vi "Quickly light intensity analyze.vi"() -> ()   [LabVIEW 2022 SP3]
uses:
  <vilib>/Math Plots/2D Math Plots/2D Compass/2D Compass XCtrl/2D Compass.xctl
  <vilib>/Analysis/7linalg.llb/Real Transpose Matrix.vi
  <vilib>/Analysis/baseanly.llb/Real A x B.vi
  <vilib>/Analysis/baseanly.llb/A x Vector.vi
  <vilib>/Utility/file.llb/Read Delimited Spreadsheet (DBL).vi
  <vilib>/Analysis/Matrix/Numeric/Conversions/Array To Matrix - RA2.vi
  <vilib>/Analysis/baseanly.llb/Real Inverse Matrix.vi
  <vilib>/Math Plots/2D Math Plots/2D Compass/2D Compass Datatype/Public/Plot Helper (Vector).vi
  <vilib>/Analysis/polynomials.llb/Polynomial Roots (DBL).vi
  <vilib>/Analysis/NI_AALPro.lvlib
  <vilib>/Math Plots/2D Math Plots/2D Compass/2D Compass Datatype/2D Compass Datatype.lvclass
  <vilib>/Math Plots/2D Math Plots/2D Plot/2D Plot Datatype/2D Plot Datatype.lvclass
  <vilib>/Analysis/Matrix/NI_Matrix.lvlib
  <vilib>/Analysis/NI_AALBase.lvlib
panel:
  in  "index":i32
  in  "Psi data base":path=path "C:/Users/User/Desktop/VASE/SiO2_70nm_Psi - 複製.txt"
  in  "Delta data base":path=path "C:/Users/User/Desktop/VASE/SiO2_70nm_Delta - 複製.txt"
  in  "VASE data index AOI35=1 ~AOI65=7":i32=2
  in  "phase retardor":dbl
  out "PSI":dbl
  out "Delta":dbl
  in  "Calculate Psi delta":bool
  out "2D Compass":refnum<class "2D Plot Datatype.lvclass">[](xcontrol)
  out "Intensity Graph 2":dbl[][](graph)
  in  "X :":dbl=1.0
  in  "Square side length:":dbl=511.0
  in  "Y :":dbl=1.0
  out "Max value(fitting)":dbl
  out "Degree exp 2":i32
  out "Max value(exp)":dbl
  in  "多項式fittng之最高次":i32=34
  in  "間隔角度":i32=10
  in  "亮度扣除基底":dbl=500.0 format="%#_13g"
  out "Intensity profile ratial":dbl
  out "all rows":dbl[][](array[numeric])
  out "Degree exp":i32
  out "Min value(exp)":dbl
  out "Min value(fitting)":dbl
  in  "起始角度":i32=10
  out "Pure Complex Roots":cdb[](array[numeric])
  out "Complex Pair Roots":cdb[](array[numeric])
  out "Seconds  2":dbl
  out "Minutes":dbl
  out "Hours  2":dbl
  out "Files currently reading  2":string
  in  "Choose an arbitrary file in the angle of incidence folder :":path
  out "極值位置":dbl[](array[numeric])
  out "Light Intensity":cluster{i32[], "Array":dbl[]}[](graph)
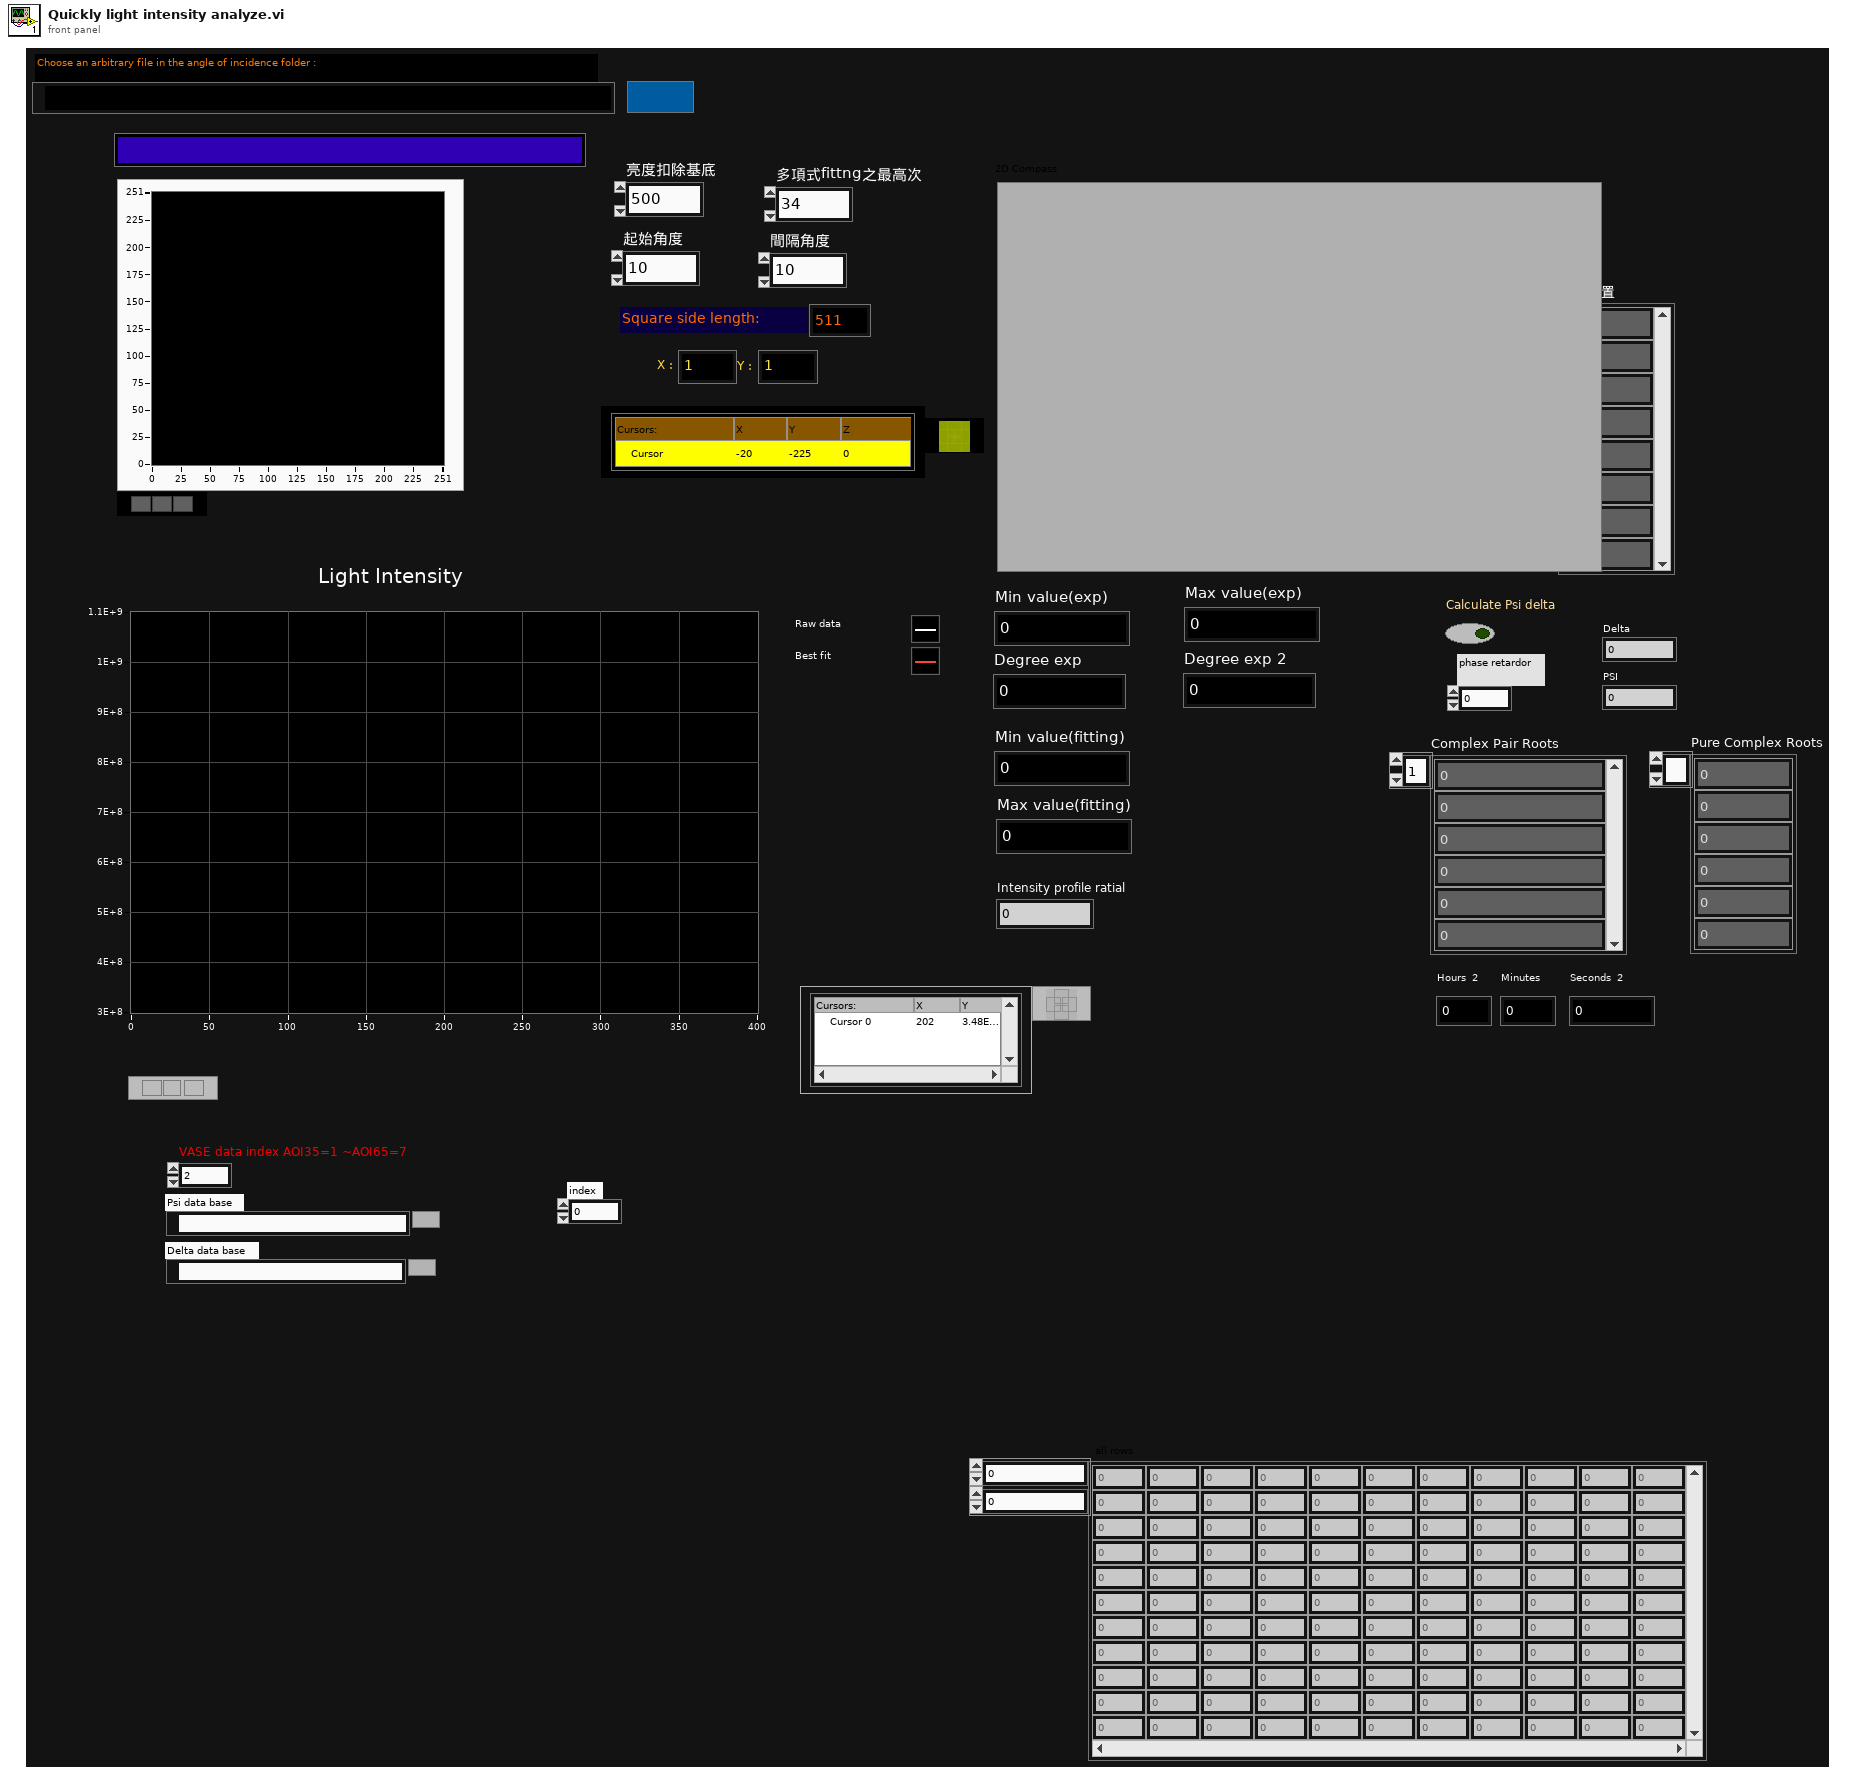
[diagram p1: front panel]
types:
  T1 = typedef "NI_Matrix.lvlib/RealMatrix.ctl" = dbl[][]
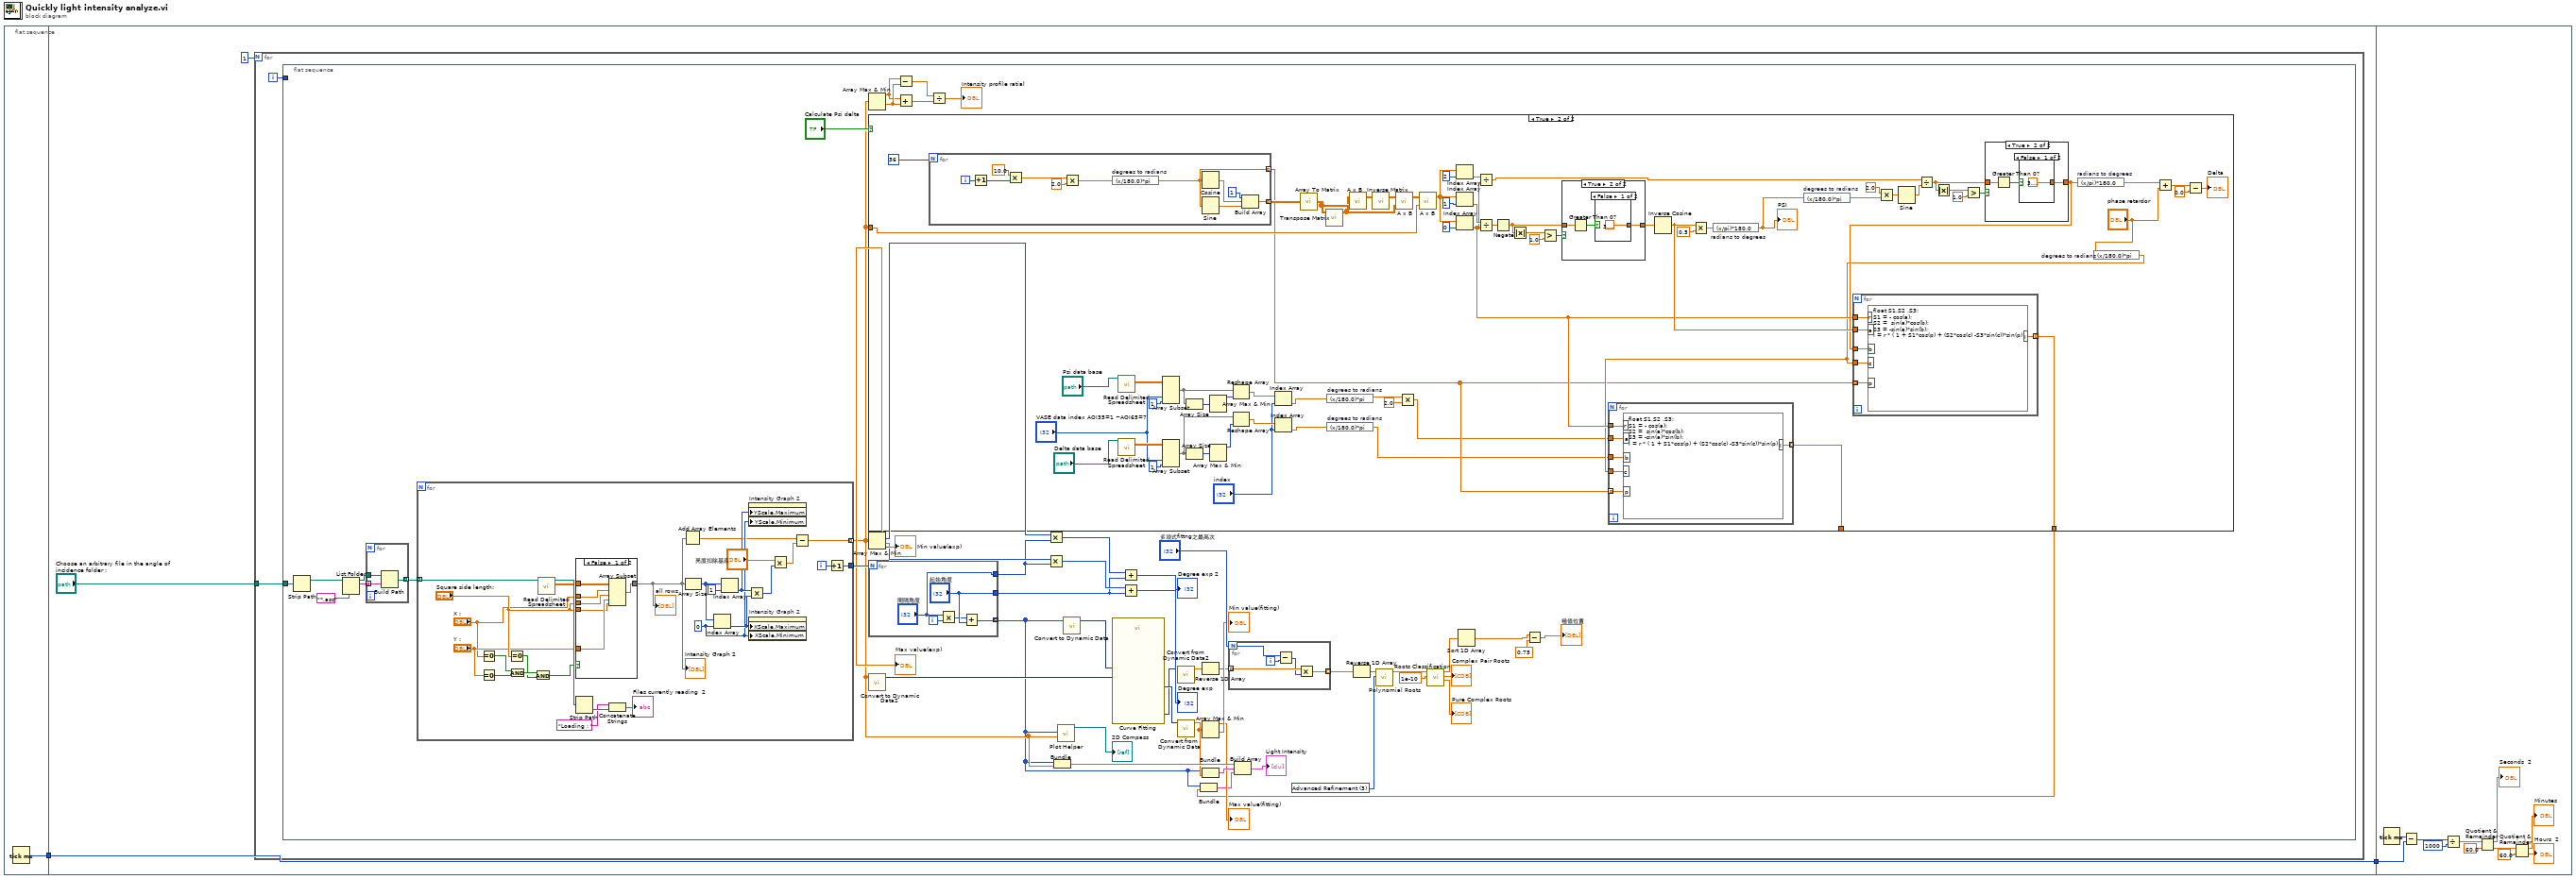
[diagram p0: block diagram]
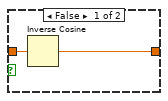
[diagram p3: hidden frame]
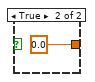
[diagram p4: hidden frame]
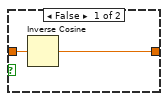
[diagram p5: hidden frame]
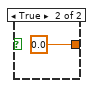
[diagram p6: hidden frame]
diagram:
  n1 = flat-sequence {
    tunnel: [w3] -> w2
    tunnel: [w6] -> w1
    tunnel: w2 -> [w6]
    tunnel: w1 -> [w211]
    frame #0 {
      n2 = Tick Count (ms)() -> (millisecond timer value=w3:u32)
    }
    frame #1 {
      n3 = for {
        N: 1 -> [_]
        tunnel: "Choose an arbitrary file in the angle of incidence folder :" -> [w7]
        i -> [w8]
        n4 = flat-sequence {
          tunnel: w8 -> [_]
          tunnel: w7 -> [w47]
          frame #0 {
            w55 = u16 3 items=["General", "Simple Classification", "Refinement", "Advanced Refinement"] ("option")
            n5 = Strip Path(path=w47) -> (stripped path=w52:path)  [unwired: 1 out]
            n6 = List Folder(path=w52, pattern="*.asc") -> (path out=w51:path, filenames=w50:string[])  [unwired: 2 in, 2 out]
            n7 = for {
              tunnel: w50 -> [w165] mode=indexing
              tunnel: w51 -> [w166]
              tunnel: [w164] -> w48 mode=indexing
              n8 = Build Path(base path=w166, name or relative path=w165) -> (appended path=w164:path)
            }
            n9 = for {
              tunnel: [w178] -> w16 mode=indexing
              tunnel: w48 -> [w199] mode=indexing
              tunnel: [w197] -> w40
              i -> [w198]
              w184 = 0 ("index")
              n10 = Equal To 0?(x="X :") -> (x = 0?=w195:bool)
              n11 = Equal To 0?(x="Y :") -> (x = 0?=w196:bool)
              n12 = Equal To 0?(x="Square side length:") -> (x = 0?=w188:bool)
              n13 = And(x=w195, y=w196) -> (x .and. y?=w194:bool)
              n14 = And(x=w194, y=w188) -> (x .and. y?=w193:bool)
              n15 = call-poly <vilib>:"Read Delimited Spreadsheet.vi"("file path (dialog if empty)"=w199) -> ("new file path (Not A Path if cancelled)"=w200:path, "all rows"=w183:dbl[][])  [unwired: 9 in, 4 out]
              n16 = case shown="False" w193 {
                tunnel: w183 -> [w209 w210]
                tunnel: "X :" -> [w207 _]
                tunnel: "Y :" -> [w206 _]
                tunnel: [w208 w210] -> w177
                tunnel: "Square side length:" -> [w205 _]
                tunnel: "Square side length:" -> [w204 _]
                frame False {
                  n17 = Array Subset(array=w209, index (row)=w207, length (row)=w205, index (col)=w206, length (col)=w204) -> (w208:dbl[][])
                }
                frame True {
                }
              }
              "all rows" <- w177
              "Intensity Graph 2" <- w177
              n18 = Strip Path(path=w200) -> (name=w202:string)  [unwired: 1 out]
              n19 = Concatenate Strings("Loading : " ("string"), w202) -> (→"Files currently reading  2":string)
              n20 = Add Array Elements(numeric array=w177) -> (sum=w182:dbl)
              n21 = Array Size(array=w177) -> (size(s)=w192:i32[])
              n22 = Index Array(array=w192, index=w184) -> (element=w189:i32)
              n23 = Index Array(array=w192, index=1) -> (element=w190:i32)
              n24 = Multiply(x=w190, y=w189) -> (x*y=w181:i32)
              n25 = property on="Intensity Graph 2" class="IntGraph (strict)"("YScale.Maximum"=w190, "YScale.Minimum"=w184) -> ()  [unwired: 2 in, 2 out]
              n26 = property on="Intensity Graph 2" class="IntGraph (strict)"("XScale.Maximum"=w189, "XScale.Minimum"=w184) -> ()  [unwired: 2 in, 2 out]
              n27 = Multiply(x="亮度扣除基底", y=w181) -> (x*y=w179:dbl)
              n28 = Subtract(x=w182, y=w179) -> (x-y=w178:dbl)
              n29 = Increment(x=w198) -> (x+1=w197:i32)
            }
            n30 = Array Max & Min(array=w16) -> (max value=w42:dbl, min value=w43:dbl)  [unwired: 2 out]
            n31 = case shown="True" "Calculate Psi delta" {
              tunnel: w16 -> [_ w112]
              tunnel: [_ w95] -> w14
              tunnel: [_ w83] -> _
              frame False {
              }
              frame True {
                n32 = for {
                  N: 36 ("Numeric") -> [_]
                  tunnel: [w160] -> w119 mode=indexing
                  tunnel: [w153] -> w84 mode=indexing
                  i -> [w163]
                  n33 = Increment(x=w163) -> (x+1=w162:i32)
                  n34 = Multiply(x=10.0, y=w162) -> (x*y=w158:dbl)
                  n35 = Multiply(x=w158, y=2.0) -> (x*y=w154:dbl)
                  n36 = expression code="(x/180.0)*pi" "degrees to radians"(w154) -> (w153:dbl)
                  n37 = Cosine(x=w153) -> (cos(x)=w156:dbl)
                  n38 = Sine(x=w153) -> (sin(x)=w157:dbl)
                  n39 = Build Array(1, w156, w157) -> (w160:dbl[])
                }
                n40 = call-poly <vilib>:"Read Delimited Spreadsheet.vi"("file path (dialog if empty)"="Psi data base") -> ("all rows"=w81:dbl[][])  [unwired: 9 in, 5 out]
                n41 = call-poly <vilib>:"Read Delimited Spreadsheet.vi"("file path (dialog if empty)"="Delta data base") -> ("all rows"=w75:dbl[][])  [unwired: 9 in, 5 out]
                n42 = Array Subset(array=w81, index (col)="VASE data index AOI35=1 ~AOI65=7", length (col)=1 ("length")) -> (w77:dbl[][])  [unwired: 2 in]
                n43 = Array Subset(array=w75, index (col)="VASE data index AOI35=1 ~AOI65=7", length (col)=1 ("length")) -> (w71:dbl[][])  [unwired: 2 in]
                n44 = Array Size(array=w77) -> (size(s)=w79:i32[])
                n45 = Array Size(array=w71) -> (size(s)=w73:i32[])
                n46 = Array Max & Min(array=w79) -> (max value=w78:i32)  [unwired: 3 out]
                n47 = Array Max & Min(array=w73) -> (max value=w72:i32)  [unwired: 3 out]
                n48 = Reshape Array(w77, w78) -> (w69:dbl[])
                n49 = Reshape Array(w71, w72) -> (w68:dbl[])
                n50 = Index Array(array=w69, index="index") -> (element=w66:dbl)
                n51 = Index Array(array=w68, index="index") -> (element=w65:dbl)
                n52 = call-poly <vilib>:"Array To Matrix.vi"("Real 2D Array"=w119) -> ("Real Matrix"=w125:T1)
                n53 = call-poly <vilib>:"Transpose Matrix.vi"("Input Matrix"=w125) -> ("Matrix Transpose"=w122:T1)  [unwired: 9 in, 1 out]
                n54 = expression code="(x/180.0)*pi" "degrees to radians"(w66) -> (w64:dbl)
                n55 = expression code="(x/180.0)*pi" "degrees to radians"(w65) -> (w61:dbl)
                n56 = call-poly <vilib>:"A x B.vi"("B"=w125, "A"=w122) -> ("A x B"=w124:T1)  [unwired: 1 out]
                n57 = call-poly <vilib>:"Inverse Matrix.vi"("Input Matrix"=w124) -> ("Inverse Matrix"=w123:T1)  [unwired: 1 in, 1 out]
                n58 = call-poly <vilib>:"A x B.vi"("B"=w122, "A"=w123) -> ("A x B"=w121:T1)  [unwired: 1 out]
                n59 = Multiply(x=w64, y=2.0) -> (x*y=w62:dbl)
                n60 = call-poly <vilib>:"A x B.vi"("Vector"=w112, "A"=w121) -> ("A x Vector"=w114:dbl[])  [unwired: 1 out]
                n61 = Index Array(array=w114, index=2) -> (element=w113:dbl)
                n62 = Index Array(array=w114, index=1) -> (element=w116:dbl)
                n63 = Index Array(array=w114, index=0) -> (element=w86:dbl)
                n64 = Divide(x=w113, y=w86) -> (x/y=w98:dbl)
                n65 = Divide(x=w116, y=w86) -> (x/y=w115:dbl)
                n66 = Negate(x=w115) -> (-x=w89:dbl)
                n67 = Absolute Value(x=w89) -> (abs(x)=w92:dbl)
                n68 = Greater?(x=w92, y=1.0) -> (0:w90:bool)
                n69 = case shown="True" w90 {
                  tunnel: [w133 w136] -> w88
                  tunnel: w89 -> [w134 w135]
                  frame False {
                    n70 = Inverse Cosine(1:w134) -> (0:w133:dbl)
                  }
                  frame True {
                    n71 = Greater Than 0?(x=w135) -> (x > 0?=w137:bool)
                    n72 = case shown="False" w137 {
                      tunnel: [3.141592653589793 0.0] -> w136
                      frame False {
                      }
                      frame True {
                      }
                    }
                  }
                }
                n73 = Inverse Cosine(1:w88) -> (0:w94:dbl)
                n74 = Multiply(x=w94, y=0.5) -> (x*y=w110:dbl)
                n75 = expression code="(x/pi)*180.0" "radians to degrees"(w110) -> (w99:dbl)
                "PSI" <- w99
                n76 = expression code="(x/180.0)*pi" "degrees to radians"(w99) -> (w104:dbl)
                n77 = Multiply(x=2.0, y=w104) -> (x*y=w102:dbl)
                n78 = Sine(x=w102) -> (sin(x)=w105:dbl)
                n79 = Divide(x=w98, y=w105) -> (x/y=w106:dbl)
                n80 = Absolute Value(x=w106) -> (abs(x)=w109:dbl)
                n81 = Greater?(x=w109, y=1.0) -> (0:w107:bool)
                n82 = case shown="True" w107 {
                  tunnel: [w146 w149] -> w93
                  tunnel: w106 -> [w147 w148]
                  frame False {
                    n83 = Inverse Cosine(1:w147) -> (0:w146:dbl)
                  }
                  frame True {
                    n84 = Greater Than 0?(x=w148) -> (x > 0?=w150:bool)
                    n85 = case shown="False" w150 {
                      tunnel: [3.141592653589793 0.0] -> w149
                      frame False {
                      }
                      frame True {
                      }
                    }
                  }
                }
                n86 = expression code="(x/pi)*180.0" "radians to degrees"(w93) -> (w101:dbl)
                n87 = expression code="(x/180.0)*pi" "degrees to radians"("phase retardor") -> (w85:dbl)
                n88 = for {
                  tunnel: w84 -> [w128] mode=indexing
                  tunnel: w86 -> [w132]
                  tunnel: w85 -> [w130]
                  tunnel: w61 -> [w131]
                  tunnel: w62 -> [w129]
                  tunnel: [w127] -> w83 mode=indexing
                  n89 = formula code="float S1,S2 ,S3;\nS1 = - cos(a);\nS2 =  sin(a)*cos(b);\nS3 = -sin(a)*sin(b);\nI = r * ( 1 + S1*cos(p) + (S2*cos(c) -S3*sin(c))*sin(p) );"("r"=w132, "a"=w129, "b"=w131, "c"=w130, "p"=w128) -> ("I"=w127:dbl)
                }
                n90 = for {
                  tunnel: w84 -> [w141] mode=indexing
                  tunnel: w86 -> [w145]
                  tunnel: w85 -> [w143]
                  tunnel: w93 -> [w144]
                  tunnel: w94 -> [w142]
                  tunnel: [w140] -> w95 mode=indexing
                  n91 = formula code="float S1,S2 ,S3;\nS1 = - cos(a);\nS2 =  sin(a)*cos(b);\nS3 = -sin(a)*sin(b);\nI = r * ( 1 + S1*cos(p) + (S2*cos(c) -S3*sin(c))*sin(p) );"("r"=w145, "a"=w142, "b"=w144, "c"=w143, "p"=w141) -> ("I"=w140:dbl)
                }
                n92 = Add(x=w101, y="phase retardor") -> (x+y=w100:dbl)
                n93 = Subtract(x=w100, y=0.0) -> (x-y=→"Delta":dbl)
              }
            }
            n94 = Array Max & Min(array=w16) -> (max value=→"Max value(exp)":dbl, max index (indices)=w34:i32, min value=→"Min value(exp)":dbl, min index (indices)=w38:i32)
            n95 = for {
              N: w40 -> [_]
              tunnel: [w176] -> w13 mode=indexing
              tunnel: ["起始角度"] -> w32
              tunnel: ["間隔角度"] -> w33
              i -> [w173]
              n96 = Multiply(x="間隔角度", y=w173) -> (x*y=w174:i32)
              n97 = Add(x=w174, y="起始角度") -> (x+y=w176:i32)
            }
            n98 = call "Convert to Dynamic Data2"("Array"=w16) -> ("Dynamic Data Type"=w26:dynamicdata)  [unwired: 3 in]
            n99 = Subtract(x=w42, y=w43) -> (x-y=w45:dbl)
            n100 = Add(x=w42, y=w43) -> (x+y=w44:dbl)
            n101 = Divide(x=w45, y=w44) -> (x/y=→"Intensity profile ratial":dbl)
            n102 = Multiply(x=w34, y=w33) -> (x*y=w35:i32)
            n103 = Multiply(x=w38, y=w33) -> (x*y=w37:i32)
            n104 = Bundle(w13, w16) -> (w56:cluster{i32[], dbl[]})  [unwired: 1 in]
            n105 = call-poly <vilib>:"Plot Helper.vi"("radius vector"=w16, "theta vector"=w13) -> ("2D Plot Class Obj Array out"=→"2D Compass":refnum<class "2D Plot Datatype.lvclass">[])  [unwired: 2 in, 7 out]
            n106 = call "Convert to Dynamic Data"("Array"=w13) -> ("Dynamic Data Type"=w27:dynamicdata)  [unwired: 3 in]
            n107 = call "Curve Fitting"("Locations"=w27, "Signals"=w26) -> ("best fit"=w25:dynamicdata, "polynomial coefficients"=w24:dynamicdata)  [unwired: 5 in, 3 out]
            n108 = Add(x=w35, y=w32) -> (x+y=→"Degree exp 2":i32)
            n109 = Add(x=w37, y=w32) -> (x+y=→"Degree exp":i32)
            n110 = call "Convert from Dynamic Data2"("Dynamic Data Type"=w24) -> ("Array"=w22:dbl[])  [unwired: 3 in]
            n111 = call "Convert from Dynamic Data"("Dynamic Data Type"=w25) -> ("Array"=w15:dbl[])  [unwired: 3 in]
            n112 = Bundle(w13, w14) -> (w12:cluster{i32[], dbl[]})  [unwired: 1 in]
            n113 = Reverse 1D Array(array=w22) -> (reversed array=w23:dbl[])
            n114 = Array Max & Min(array=w15) -> (max value=→"Max value(fitting)":dbl, min value=→"Min value(fitting)":dbl)  [unwired: 2 out]
            n115 = Bundle(w13, "Array"=w15) -> (w58:cluster{i32[], "Array":dbl[]})  [unwired: 1 in]
            n116 = for {
              N: "多項式fittng之最高次" -> [w168]
              tunnel: w23 -> [w171] mode=indexing
              tunnel: [w167] -> w21 mode=indexing
              i -> [w169]
              n117 = Subtract(x=w168, y=w169) -> (x-y=w170:i32)
              n118 = Multiply(x=w171, y=w170) -> (x*y=w167:dbl)
            }
            n119 = Build Array(w56, w58, w12) -> (→"Light Intensity":cluster{i32[], "Array":dbl[]}[])
            n120 = Reverse 1D Array(array=w21) -> (reversed array=w20:dbl[])
            n121 = call-poly <vilib>:"Polynomial Roots.vi"("option"=w55, "P(x)"=w20) -> ("Roots"=w59:cdb[])  [unwired: 8 in, 1 out]
            n122 = call <vilib>:"Roots Classification.vi"("tolerance for real roots"=1e-10, "Roots"=w59) -> ("Pure Complex Roots"=→"Pure Complex Roots":cdb[], "Complex Pair Roots"=→"Complex Pair Roots":cdb[], "Real Roots"=w60:dbl[])  [unwired: 6 in, 1 out]
            n123 = Sort 1D Array(array=w60) -> (sorted array=w11:dbl[])
            n124 = Subtract(x=w11, y=0.75) -> (x-y=→"極值位置":dbl[])
          }
        }
      }
    }
    frame #2 {
      n125 = Tick Count (ms)() -> (millisecond timer value=w218:u32)
      n126 = Subtract(x=w218, y=w211) -> (x-y=w219:u32)
      n127 = Divide(x=w219, y=u32 1000) -> (x/y=w220:dbl)
      n128 = Quotient & Remainder(x=w220, y=60.0) -> (x-y*floor(x/y)=→"Seconds  2":dbl, floor(x/y)=w221:dbl)
      n129 = Quotient & Remainder(x=w221, y=60.0) -> (x-y*floor(x/y)=→"Minutes":dbl, floor(x/y)=→"Hours  2":dbl)
    }
  }
